vi "configure.vi"(8 "error in (no error)":errorcluster, 11 "TrajectoryDL110420DoubleCircle.lvclass in":refnum<class "TrajectoryDL110420DoubleCircle.lvclass">) -> (0 "error out":errorcluster, 3 "TrajectoryDL110420DoubleCircle.lvclass 2 out":refnum<class "TrajectoryDL110420DoubleCircle.lvclass">)   [LabVIEW 2010, in "TrajectoryDL110420DoubleCircle.lvclass"]
doc: "The dynamic dispatch version of this VI loads and displays the configuration file associated with the plug-in object. The user modify and save the configuration data."
uses:
  TrajectoryDL110420DoubleCircle.lvclass
  center_type_enum.ctl
  TrajectoryDL110420DoubleCircle.lvclass/TrajectoryDL110420DoubleCircle.ctl
  common/classes/GenericComponent/GenericComponent/GenericComponent.lvclass
panel:
  in  "center type":T1
  in  "z offset XPath":string caption="z offset"
  in  "y offset XPath":string caption="y offset"
  in  "x offset XPath":string caption="x offset"
  out "configuration":string
  in  "cancelButton":bool
  in  "okButton":bool
  # "Configure TrajectoryDL110420DoubleCircle"
  # "XPaths"
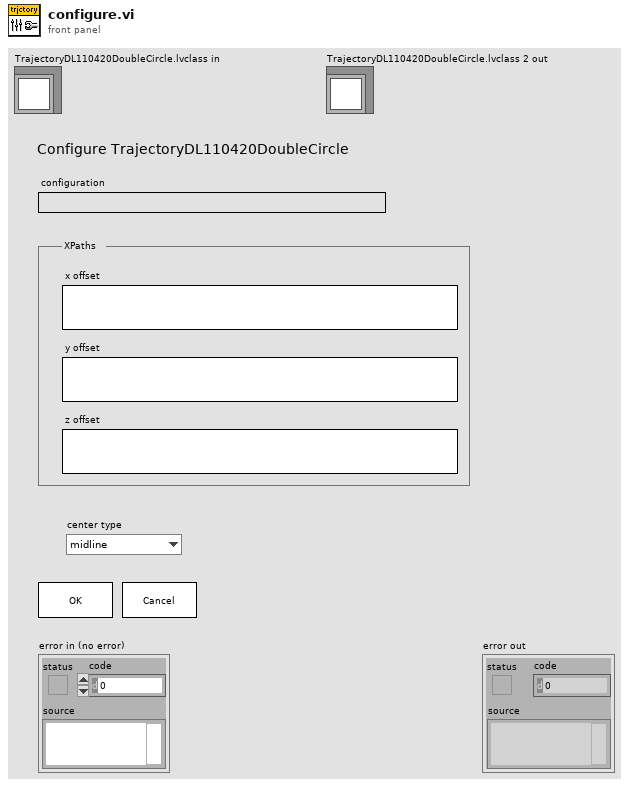
[diagram p1: front panel]
types:
  T1 = typedef "center_type_enum.ctl" = enum16{"midline", "centroid"}
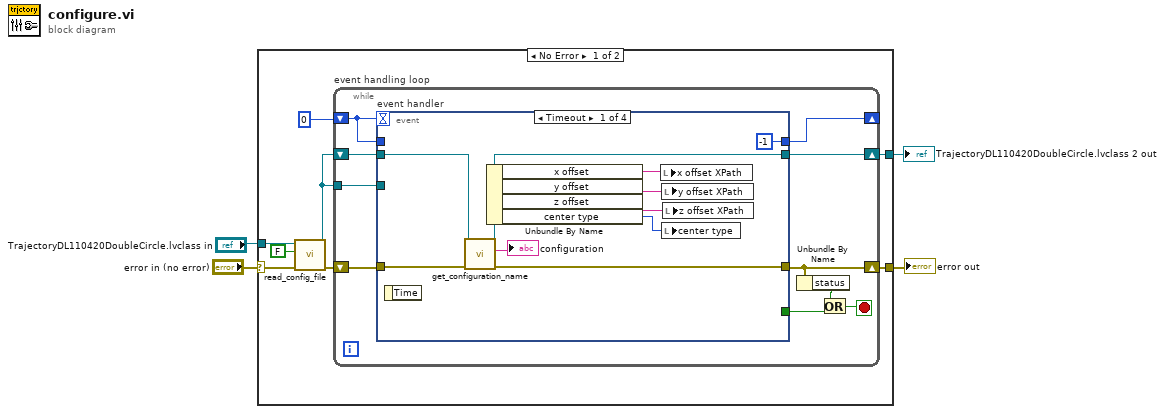
[diagram p0: block diagram]
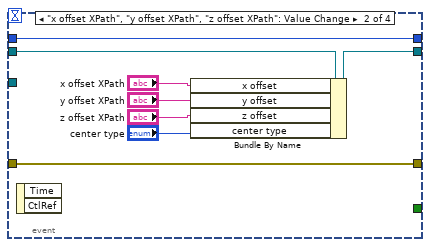
[diagram p2: hidden frame]
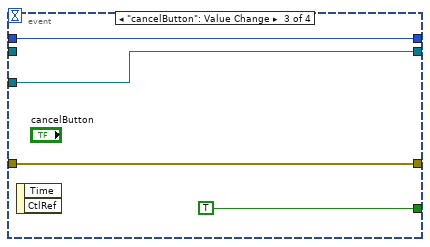
[diagram p3: hidden frame]
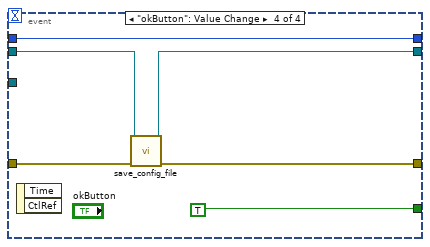
[diagram p4: hidden frame]
diagram:
  n1 = case shown="No Error" "error in (no error)" {
    selector: "error in (no error)" -> [w9 w52]
    tunnel: "TrajectoryDL110420DoubleCircle.lvclass in" -> [w7 w51]
    tunnel: [w11 w52] -> w3
    tunnel: [w12 w51] -> w2
    frame No Error {
      n2 = call-dynamic "read_config_file.vi"("error in (no error)"=w9, "force load?"=FALSE, "GenericPlugin in"=w7) -> ("error out"=w8:errorcluster, "GenericPlugin out"=w6:refnum<class "TrajectoryDL110420DoubleCircle.lvclass">)  [unwired: 7 in]
      n3 = while "event handling loop" {
        shift-right: [w20] -> w12
        shift-left: w6 -> [w22]
        shift-right: [w19] -> w11
        shift-left: w8 -> [w21]
        shift-right: [w14] -> _
        shift-left: 0 -> [w15]
        tunnel: w6 -> [w13]
        stop <- w16 stop-if-true
        n4 = event "event handler" shown="[0] Timeout" {
          selector: _ -> [_ _ _ _]
          dyn-events: _ -> [_ _ _ _]
          timeout: w15 -> [_ _ _ _]
          tunnel: w22 -> [w32 w34 _ w46]
          tunnel: w21 -> [w30 w40 w44 w48]
          tunnel: [w29 w40 w44 w47] -> w19
          tunnel: [w31 w33 w41 w45] -> w20
          tunnel: [_ _ TRUE TRUE] -> w18
          tunnel: [-1 w39 w42 w49] -> w14
          tunnel: w15 -> [_ w39 w42 w49]
          tunnel: w13 -> [_ _ w41 _]
          event Timeout {
            n5 = event-data() -> ()  [unwired: 1 in, 1 out]
            n6 = call "get_configuration_name.vi"("error in (no error)"=w30, "GenericPlugin.lvclass in"=w32) -> ("error out"=w29:errorcluster, "configuration name"=→"configuration":string, "GenericPlugin.lvclass out"=w31:refnum<class "TrajectoryDL110420DoubleCircle.lvclass">)  [unwired: 7 in]
            n7 = Unbundle By Name(w31) -> ("x offset"=w27:string, "y offset"=w25:string, "z offset"=w26:string, "center type"=w24:T1)
            n8 = local write "x offset XPath"(w27) -> ()
            n9 = local write "y offset XPath"(w25) -> ()
            n10 = local write "center type"(w24) -> ()
            n11 = local write "z offset XPath"(w26) -> ()
          }
          event "x offset XPath", "y offset XPath", "z offset XPath": Value Change {
            n12 = event-data() -> ()  [unwired: 1 in, 2 out]
            n13 = Bundle By Name(cluster=w34, "x offset"="x offset XPath", "y offset"="y offset XPath", "z offset"="z offset XPath", "center type"="center type") -> (w33:refnum<class "TrajectoryDL110420DoubleCircle.lvclass">)
          }
          event "cancelButton": Value Change {
            n14 = event-data() -> ()  [unwired: 1 in, 2 out]
          }
          event "okButton": Value Change {
            n15 = event-data() -> ()  [unwired: 1 in, 2 out]
            n16 = call-dynamic "save_config_file.vi"("error in (no error)"=w48, "GenericPlugin in"=w46) -> ("error out"=w47:errorcluster, "GenericPlugin out"=w45:refnum<class "TrajectoryDL110420DoubleCircle.lvclass">)  [unwired: 8 in]
          }
        }
        n17 = Unbundle By Name(w19) -> ("status"=w17:bool)
        n18 = Or(x=w17, y=w18) -> (x .or. y?=w16:bool)
      }
    }
    frame Error {
    }
  }
  "error out" <- w3
  "TrajectoryDL110420DoubleCircle.lvclass 2 out" <- w2
